vi "Team Stats.vi"(11 "Team":refnum<class "Team.lvclass">) -> (2 "Team Stats":T1)   [LabVIEW 2020, in "SquareBattle.lvlib" / "Team.lvclass"]
doc: "Provides the current team stats, which are updated at the end of each round. This provides a count of the:\n\n - active squares on your team\n - number of squares that have been replicated this game (including the starting square)\n - the number of other teams' squares that your team has killed\n - the count of your squares that have been attacked by other teams\n - how many collisions from any team that have resulted in your squares being lost"
uses:
  Team.lvclass
  Team Stats.ctl
  Team.lvclass/Team.ctl
  SquareBattle.lvlib
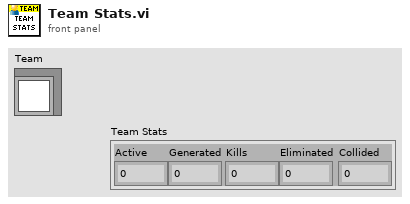
[diagram p1: front panel]
types:
  T1 = typedef "SquareBattle.lvlib/Team Stats.ctl" = cluster{"Active":i32, "Generated":i32, "Kills":i32, "Eliminated":i32, "Collided":i32}
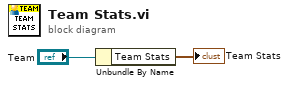
[diagram p0: block diagram]
diagram:
  n1 = Unbundle By Name("Team") -> ("Team Stats"=→"Team Stats":T1)
